vi "filter_wash_data.vi"(6 "timeout (25000ms)":i32=25000, 8 "error in (no error)":errorcluster, 11 "daemon reference in":refnum<k5>) -> (0 "error out":errorcluster, 1 "filter_wash_debug_data":T1, 2 "response":string, 3 "daemon reference out":refnum<k5>, 5 "command out":string="random")   [LabVIEW 2017]
doc: "<b>Command: </b>\"filter_wash_data\"\n\n<b>Description: </b> This command will get related datas from filter wash for tesing, collecting data values.\n\n<b>Parameters: </b> None\nField |Type |Size |Offset | Units | Description\ndeltaP_Pa | Signed Integer |4 | 0 |Pa | Delta | pressure in Pa\nshaftPower_mW Signed Integer 4 4 mW shaft power in mW\nambientP_Pa Signed Integer 4 8 Pa ambient pressure in Pa\ncurrentP_Pa Signed Integer 4 12 Pa running pressure in Pa\nambientTemp_mC Signed Integer 4 16 Pa ambient temperature in C\nnormDeltaP_mPa Signed Integer 4 20 mPa normalised delta pressure in milli- -Pa, divide 1000 to get Pa\n\n\nnormDeltaPfiltered_mPa Signed Integer 4 24 mPa filtered normalised delta pressure in\nmilli-Pa, divide 1000 to get Pa\n\nfitlerWashThreshold Signed Integer 4 28 mPa filtered wash threshold in milli-Pa or\nmilli-rpm, divide 1000 to get Pa or rpm\n\nspeed_rpm Signed Integer 4 32 rpm motor speed\nnormSpeed_mrpm Signed Integer 4 36 mrpm normalised motor speed in milli-rpm\n,divide 1000 to get rpm.\n\nnormSpeedFiltered_mrpm Signed Integer 4 40 mrpm filtered normalised motor speed in milli-rpm ,divide 1000 to get rpm.\n\n____________________________________________\nDIPC 692 Daemon API 10.0.0.1\nSam Tee - Dyson Technology Ltd\nCopyright (c) 2024, Dyson Technology Ltd"
uses:
  typdef/filter_wash_debug_data.ctl
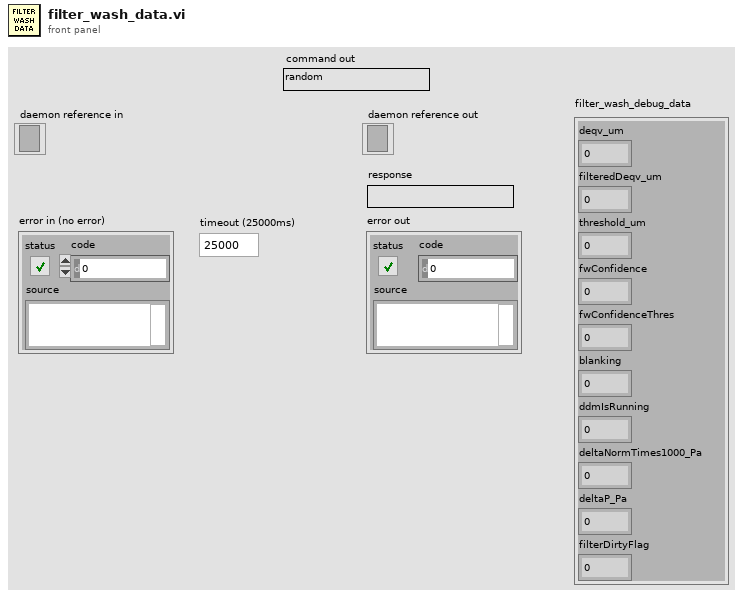
[diagram p1: front panel]
types:
  T1 = typedef "filter_wash_debug_data.ctl" = cluster{"deqv_um":dbl, "filteredDeqv_um":dbl, "threshold_um":dbl, "fwConfidence":dbl, "fwConfidenceThres":dbl, "blanking":dbl, "ddmIsRunning":dbl, "deltaNormTimes1000_Pa":dbl, "deltaP_Pa":dbl, "filterDirtyFlag":dbl}
  T2 = cluster{"array type (2D Dbl)[0]":dbl, "array type (2D Dbl)[1]":dbl, "array type (2D Dbl)[2]":dbl, "array type (2D Dbl)[3]":dbl, "array type (2D Dbl)[4]":dbl, "array type (2D Dbl)[5]":dbl, "array type (2D Dbl)[6]":dbl, "array type (2D Dbl)[7]":dbl, "array type (2D Dbl)[8]":dbl, "array type (2D Dbl)[9]":dbl}
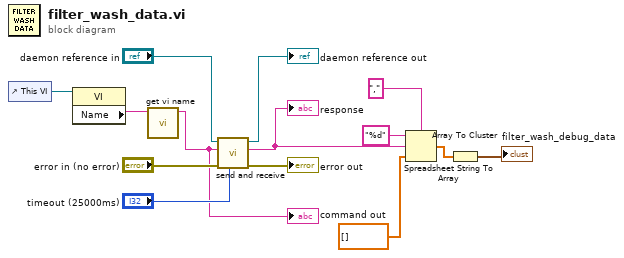
[diagram p0: block diagram]
diagram:
  n1 = control-ref of="This VI"() -> (w9:refnum<vi>)
  n2 = property class="VI"(reference=w9) -> ("Name"=w8:string)  [unwired: 1 in, 2 out]
  n3 = call "get vi name.vi"("library.lvlib:name.vi"=w8) -> ("vi name"=w7:string)  [unwired: 10 in]
  "command out" <- w7
  n4 = call "send and receive.vi"("timeout (25000ms)"="timeout (25000ms)", "error in (no error)"="error in (no error)", "command"=w7, "daemon reference in"="daemon reference in") -> ("error out"=→"error out":errorcluster, "response"=w6:string, "daemon reference out"=→"daemon reference out":refnum<k5>)  [unwired: 5 in]
  "response" <- w6
  n5 = Spreadsheet String To Array(delimiter (Tab)=",", format string="%d", spreadsheet string=w6, array type (2D Dbl)=dbl[] []) -> (array=w3:dbl[])
  n6 = Array To Cluster(array=w3) -> (cluster=→"filter_wash_debug_data":T2)
